vi "Monitor.vi"() -> ()   [LabVIEW 2015]
uses:
  Libraries/NI-DAQ/NI-DAQ digitizer parameters.ctl
  Libraries/File/Controls/File formats.ctl
panel:
  out "Shot data":string
  out "file path out":path
  out "Waveform Graph":waveform(dbl)[](graph)
  in  "Shots file":path=path "Y:/ShotHistory2016.txt"
  in  "Log file folder":path=path "C:/Data"
  out "Match out":errorcluster
  out "new path":path
  in  "Root Data Folder":path=path "C:/Data/idot"
  out "File count":i32
  out "New data file event":path
  out "Final error out":errorcluster
  out "Recorder Error Out":errorcluster
  in  "Parameters":T1={"physical channels"="Dev1/ai0:7", "input terminal configuration"=10106, "Range"=10.0, "Sample rate"=1000000.0, "samples per channel"=102400, "Trigger source"="/Dev1/PFI0", "pretrigger samples per channel"=1000, "task"="", "Sample mode"=10178, "Retriggerable"=FALSE, "File Path"=path "C:/Data/idot/test.tdms"} {"Sample mode" items=["Finite Samples"=10178, "Continuous Samples"=10123, "Hardware Timed Single Point"=12522]; "samples per channel" format="%d (0x%x)"; "Sample rate" format="%.2p"; "input terminal configuration" items=["default"=-1, "RSE"=10083, "NRSE"=10078, "Differential"=10106, "Pseudodifferential"=12529]}
  in  "Process Stop Button":bool
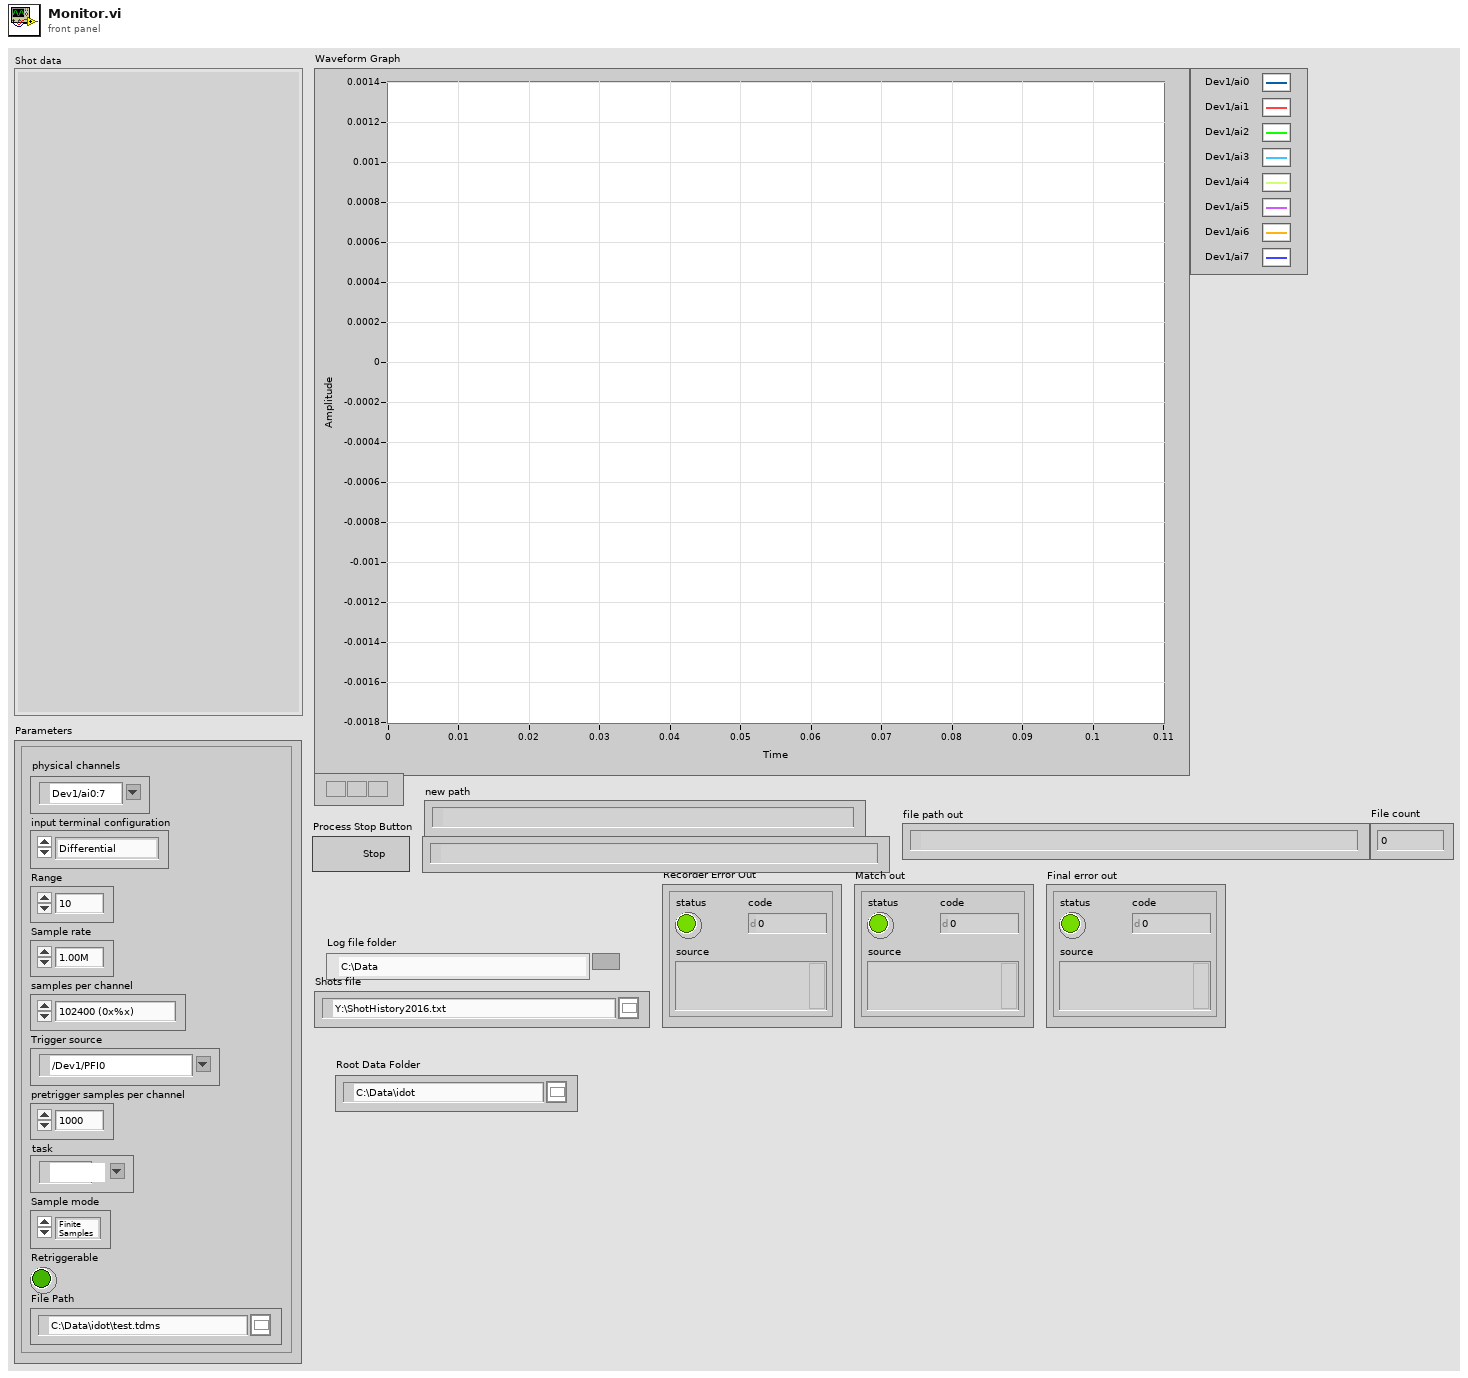
[diagram p1: front panel]
types:
  T1 = typedef "NI-DAQ digitizer parameters.ctl" = cluster{"physical channels":tag, "input terminal configuration":i32, "Range":dbl, "Sample rate":dbl, "samples per channel":i32, "Trigger source":tag, "pretrigger samples per channel":u32, "task":refnum<k21>, "Sample mode":i32, "Retriggerable":bool, "File Path":path}
  T2 = enum16{"open", "open or create", "create or replace", "create", "open (read-only)"}
  T3 = typedef "File formats.ctl" = enum16{"TDMS", "ASCII", "BINARY"}
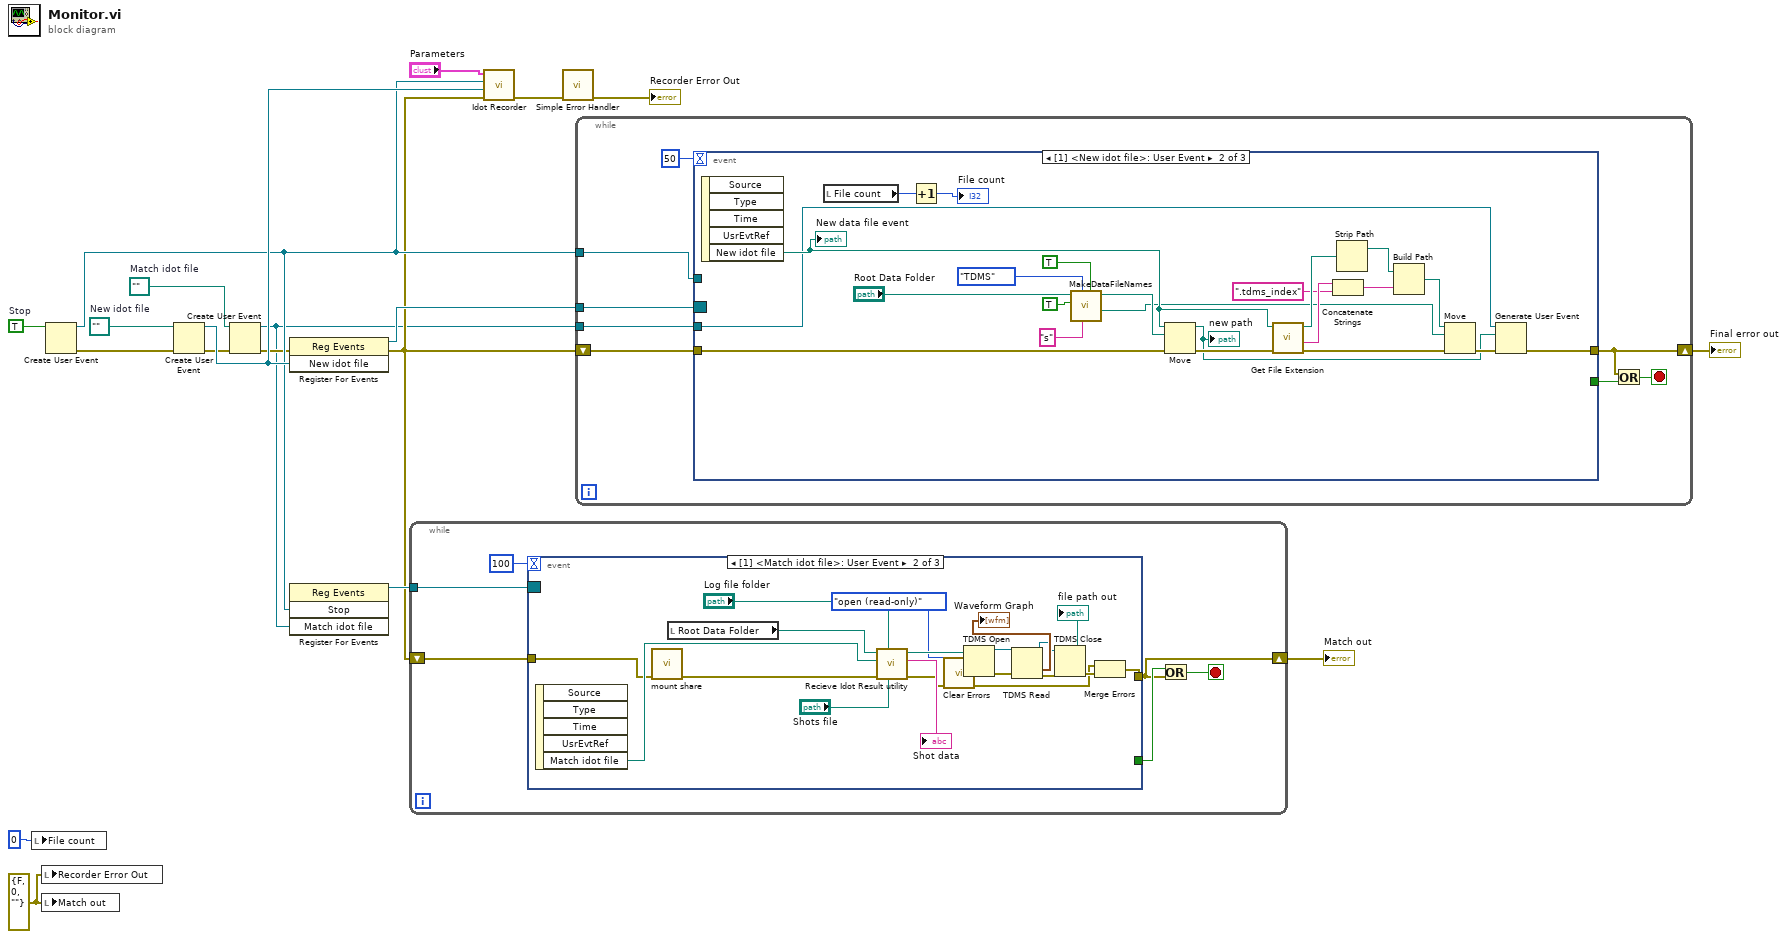
[diagram p0: block diagram]
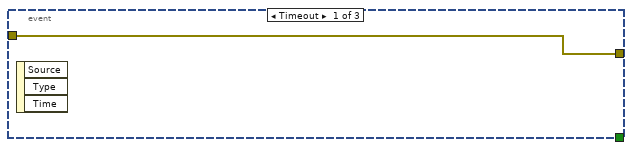
[diagram p2: hidden frame]
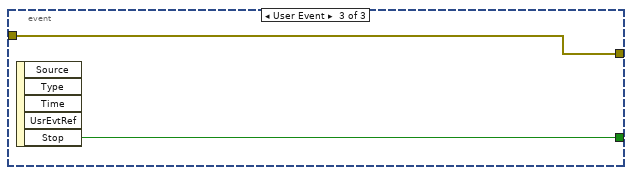
[diagram p3: hidden frame]
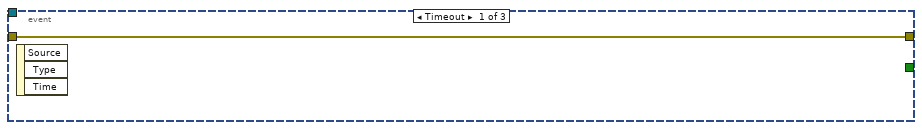
[diagram p4: hidden frame]
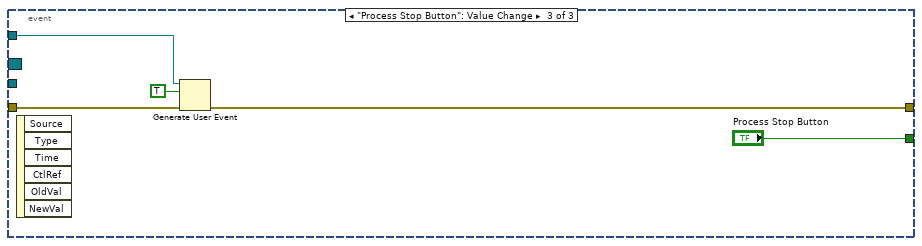
[diagram p5: hidden frame]
diagram:
  w6 = path ""  # Match idot file
  w2 = errorcluster {"status"=FALSE, "code"=0, "source"=""} ("Recorder Error Out")
  w18 = path ""  # New idot file
  w19 = TRUE  # Stop
  n1 = local write "File count"(0) -> ()
  n2 = local write "Recorder Error Out"(w2) -> ()
  n3 = local write "Match out"(w2) -> ()
  n4 = Create User Event(user event datatype=w19) -> (user event=w9:refnum<user-event>, error out=w16:errorcluster)  [unwired: 1 in]
  n5 = Create User Event(user event datatype=w18, error in=w16) -> (user event=w14:refnum<user-event>, error out=w8:errorcluster)
  n6 = Create User Event(user event datatype=w6, error in=w8) -> (user event=w1:refnum<user-event>, error out=w7:errorcluster)
  n7 = register-events(error in=w7, w14) -> (reference out=w13:refnum<event-registration>, error out=w4:errorcluster)  [unwired: 1 in]
  n8 = register-events(w9, w1) -> (reference out=w5:refnum<event-registration>)  [unwired: 2 in, 1 out]
  n9 = while {
    tunnel: w5 -> [w24]
    shift-right: [w20] -> w3
    shift-left: w4 -> [w22]
    stop <- w21 stop-if-true
    n10 = event shown="[1] <Match idot file>: User Event" {
      selector: w24 -> [_ _ _]
      dyn-events: _ -> [_ _ _]
      timeout: 100 -> [_ _ _]
      tunnel: [_ _ w47] -> w23
      tunnel: w22 -> [w26 w41 w46]
      tunnel: [w26 w29 w46] -> w20
      event Timeout {
        n11 = event-data() -> ()  [unwired: 1 in, 3 out]
      }
      event User Event {
        n12 = event-data() -> ("Match idot file"=w45:path)  [unwired: 1 in, 4 out]
        n13 = call "mount share.vi"("Error In"=w41) -> ("Error Out"=w40:errorcluster)  [unwired: 9 in, 1 out]
        n14 = local read "Root Data Folder"() -> (w44:path)
        n15 = call "Recieve Idot Result utility.vi"("Shots file"="Shots file", "Log file folder"="Log file folder", "error in (no error)"=w40, "file path"=w45, "Root Data Folder"=w44) -> ("error out"=w28:errorcluster, "Formated shot data"=→"Shot data":string, "File Path output"=w39:path)  [unwired: 4 in]
        n16 = call <vilib>:"Clear Errors.vi"("error in (no error)"=w28) -> ("error out"=w27:errorcluster)  [unwired: 5 in, 1 out]
        n17 = TDMS Open(10:T2."open (read-only)" ("operation (0:open)"), 11:w39) -> (0:w36:errorcluster, 3:w37:refnum<k34>)  [unwired: 5 in]
        n18 = TDMS Read(0:w37, 11:w36) -> (4:w32:refnum<k34>, 10:→"Waveform Graph":waveform(dbl)[], 15:w34:errorcluster)  [unwired: 6 in, 3 out]
        n19 = TDMS Close(8:w34, 11:w32) -> (0:w33:errorcluster, 3:→"file path out":path)
        n20 = Merge Errors(w27, w33) -> (w29:errorcluster)
      }
      event User Event {
        n21 = event-data() -> ("Stop"=w47:bool)  [unwired: 1 in, 4 out]
      }
    }
    n22 = Or(x=w23, y=w20) -> (x .or. y?=w21:bool)
  }
  "Match out" <- w3
  n23 = call "Idot Recorder.vi"("Error In"=w4, "New idot file event"=w14, "Stop event"=w9, "Parameters"="Parameters") -> ("Error Out"=w15:errorcluster)  [unwired: 7 in]
  n24 = call <vilib>:"Simple Error Handler.vi"("error in (no error)"=w15) -> ("error out"=→"Recorder Error Out":errorcluster)  [unwired: 4 in, 4 out]
  n25 = while {
    tunnel: w13 -> [w54]
    shift-right: [w50] -> w12
    shift-left: w4 -> [w52]
    tunnel: w9 -> [w53]
    tunnel: w1 -> [w48]
    stop <- w51 stop-if-true
    n26 = event shown="[1] <New idot file>: User Event" {
      selector: w54 -> [_ _ _]
      dyn-events: _ -> [_ _ _]
      timeout: 50 -> [_ _ _]
      tunnel: [_ _ "Process Stop Button"] -> w55
      tunnel: w53 -> [_ _ w83]
      tunnel: w52 -> [w56 w71 w82]
      tunnel: [w56 w59 w81] -> w50
      tunnel: w48 -> [_ w58 _]
      event Timeout {
        n27 = event-data() -> ()  [unwired: 1 in, 3 out]
      }
      event User Event {
        n28 = event-data() -> ("New idot file"=w70:path)  [unwired: 1 in, 4 out]
        "New data file event" <- w70
        n29 = local read "File count"() -> (w78:i32)
        n30 = Increment(x=w78) -> (x+1=→"File count":i32)
        n31 = call "MakeDataFileNames.vi"("Include time"=TRUE, "File Prefix"="s", "File format"=File_formats."TDMS", "Generate Index"=TRUE, "Root Data Folder"="Root Data Folder") -> ("Index  File Path"=w61:path, "Data File  Path"=w72:path)  [unwired: 3 in, 2 out]
        n32 = Move(source path=w70, error in=w71, 10:w72) -> (error out=w64:errorcluster, 3:w57:path)  [unwired: 2 in, 1 out]
        "new path" <- w57
        n33 = call <vilib>:"Get File Extension.vi"("error in (no error)"=w64, "file"=w70) -> ("error out"=w63:errorcluster, "filename without extension"=w67:string, "dup file"=w69:path)  [unwired: 5 in, 2 out]
        n34 = Concatenate Strings(w67, ".tdms_index" ("string")) -> (w65:string)
        n35 = Strip Path(path=w69) -> (stripped path=w68:path)  [unwired: 1 out]
        n36 = Build Path(base path=w68, name or relative path=w65) -> (appended path=w62:path)
        n37 = Move(source path=w62, error in=w63, 10:w61) -> (error out=w60:errorcluster)  [unwired: 2 in, 2 out]
        n38 = Generate User Event(user event=w58, event data cluster=w57, error in=w60) -> (error out=w59:errorcluster)  [unwired: 1 in, 1 out]
      }
      event "Process Stop Button": Value Change {
        n39 = event-data() -> ()  [unwired: 1 in, 6 out]
        n40 = Generate User Event(user event=w83, event data cluster=TRUE ("event data"), error in=w82) -> (error out=w81:errorcluster)  [unwired: 1 in, 1 out]
      }
    }
    n41 = Or(x=w50, y=w55) -> (x .or. y?=w51:bool)
  }
  "Final error out" <- w12
